vi "Set Name.vi"(10 "name":string, 11 "Component in":refnum<class "Component.lvclass">) -> (3 "Component out":refnum<class "Component.lvclass">)   [LabVIEW 2019, in "DSF Core.lvlib" / "Component.lvclass"]
uses:
  Component.lvclass
  Component.lvclass/Component.ctl
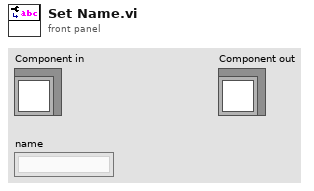
[diagram p1: front panel]
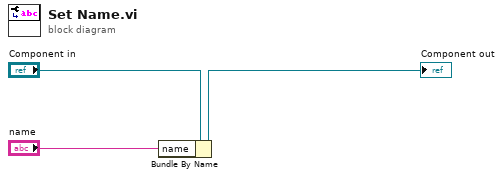
[diagram p0: block diagram]
diagram:
  n1 = Bundle By Name(cluster="Component in", "name"="name") -> (→"Component out":refnum<class "Component.lvclass">)
